vi "Supports Folder.vi"(8 "error in (no error)":errorcluster, 10 "Folder":path, 11 "NamedPackage in":refnum<class "NamedPackage.lvclass">) -> (0 "error out":errorcluster, 1 "Root Folder":path, 2 "Supported":bool, 3 "NamedPackage out":refnum<class "NamedPackage.lvclass">)   [LabVIEW 2020, in "GPack.lvlib" / "NamedPackage.lvclass"]
uses:
  NamedPackage.lvclass
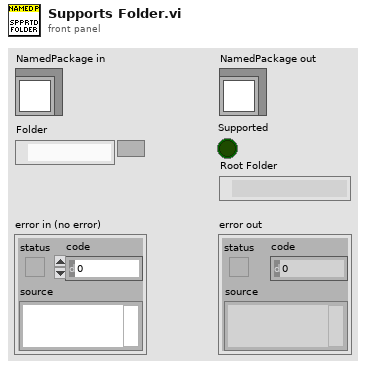
[diagram p1: front panel]
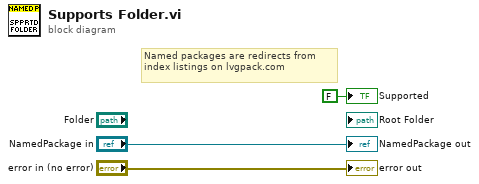
[diagram p0: block diagram]
diagram:
  # "Named packages are redirects from index listings on lvgpack.com"
  "error out" <- "error in (no error)"
  "NamedPackage out" <- "NamedPackage in"
  "Supported" <- FALSE ("Supported")
